vi "DHE_TPs2DArrr.vi"(10 "TPs":T1[](array[typedef]) {"Limits"."nominal" format="%.2f"; "Limits"."Lower" format="%.2f"; "Limits"."upper" format="%.2f"}) -> (2 "TPs out":string[][](table))   [LabVIEW 2016]
uses:
  DHE_TP.ctl
  DHE_TPLimits.ctl
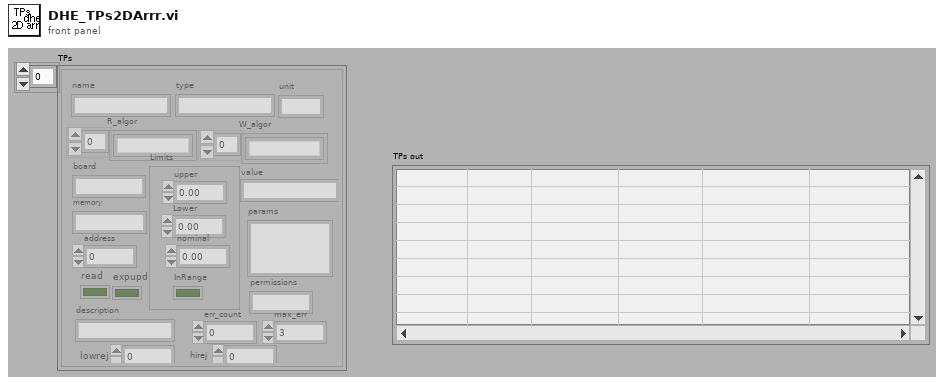
[diagram p1: front panel]
types:
  T1 = typedef "DHE_TP.ctl" = cluster{"name":string, "type":string, "R_algor":string[], "board":string, "memory":string, "address":i32, "value":string, "Limits":T2, "unit":string, "params":string, "permissions":string, "W_algor":string[], "description":string, "err_count":i32, "max_err":i32, "read":bool, "lowrej":dbl, "hirej":dbl, "expupd":bool}
  T2 = typedef "DHE_TPLimits.ctl" = cluster{"upper":dbl, "Lower":dbl, "InRange":bool, "nominal":dbl}
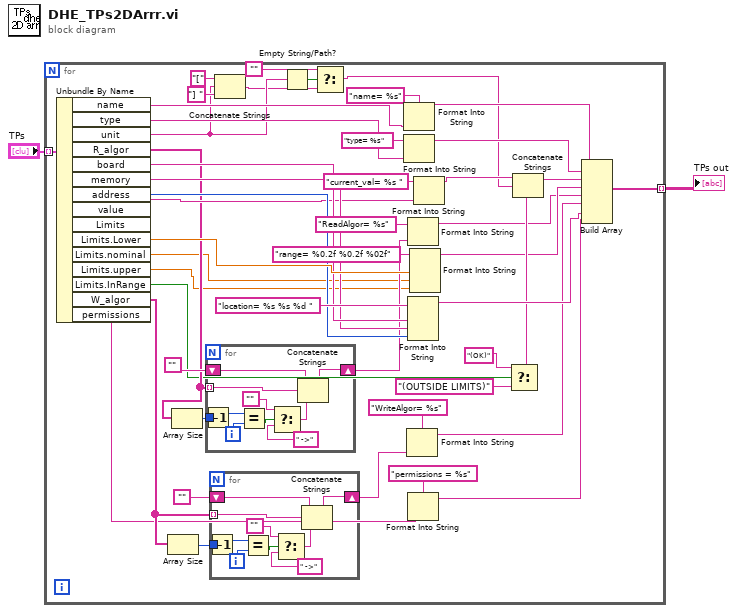
[diagram p0: block diagram]
diagram:
  n1 = for {
    tunnel: "TPs" -> [w50] mode=indexing
    tunnel: [w33] -> w1 mode=indexing
    n2 = Unbundle By Name(w50) -> ("name"=w48:string, "type"=w46:string, "unit"=w21:string, "R_algor"=w31:string[], "board"=w41:string, "memory"=w40:string, "address"=w39:i32, "value"=w37:string, "Limits.Lower"=w43:dbl, "Limits.nominal"=w4:dbl, "Limits.upper"=w5:dbl, "Limits.InRange"=w19:bool, "W_algor"=w12:string[], "permissions"=w7:string)  [unwired: 1 out]
    n3 = Array Size(array=w12) -> (size(s)=w13:i32)
    n4 = Array Size(array=w31) -> (size(s)=w30:i32)
    n5 = for {
      tunnel: w31 -> [w70] mode=indexing
      shift-right: [w69] -> w29
      shift-left: "" -> [w68]
      tunnel: w30 -> [w67]
      i -> [w66]
      n6 = Decrement(x=w67) -> (x-1=w61:i32)
      n7 = Equal?(x=w61, y=w66) -> (x = y?=w65:bool)
      n8 = Select(t="", s=w65, f=" ->") -> (s? t:f=w62:string)
      n9 = Concatenate Strings(w68, w70, w62) -> (w69:string)
    }
    n10 = for {
      tunnel: w12 -> [w60] mode=indexing
      shift-right: [w59] -> w10
      shift-left: "" -> [w58]
      tunnel: w13 -> [w57]
      i -> [w56]
      n11 = Decrement(x=w57) -> (x-1=w51:i32)
      n12 = Equal?(x=w51, y=w56) -> (x = y?=w55:bool)
      n13 = Select(t="", s=w55, f=" ->") -> (s? t:f=w52:string)
      n14 = Concatenate Strings(w58, w60, w52) -> (w59:string)
    }
    n15 = Concatenate Strings("[" ("string"), w21, "] " ("string")) -> (w20:string)
    n16 = Empty String/Path?(string/path=w21) -> (empty?=w28:bool)
    n17 = Select(t="", s=w28, f=w20) -> (s? t:f=w25:string)
    n18 = Format Into String(format string="name= %s", w48) -> (resulting string=w36:string)  [unwired: 2 in, 1 out]
    n19 = Format Into String(format string="type= %s", w46) -> (resulting string=w35:string)  [unwired: 2 in, 1 out]
    n20 = Format Into String(format string="WriteAlgor= %s", w10) -> (resulting string=w9:string)  [unwired: 2 in, 1 out]
    n21 = Format Into String(format string="ReadAlgor= %s", w29) -> (resulting string=w14:string)  [unwired: 2 in, 1 out]
    n22 = Format Into String(format string="location= %s %s %d ", w41, w40, w39) -> (resulting string=w34:string)  [unwired: 2 in, 1 out]
    n23 = Format Into String(format string="permissions = %s", w7) -> (resulting string=w6:string)  [unwired: 2 in, 1 out]
    n24 = Format Into String(format string="range= %0.2f %0.2f %02f", w43, w4, w5) -> (resulting string=w15:string)  [unwired: 2 in, 1 out]
    n25 = Format Into String(format string="current_val= %s ", w37) -> (resulting string=w26:string)  [unwired: 2 in, 1 out]
    n26 = Select(t="(OK)", s=w19, f="(OUTSIDE LIMITS)") -> (s? t:f=w16:string)
    n27 = Concatenate Strings(w26, w25, w16) -> (w24:string)
    n28 = Build Array(w36, w35, w24, w15, w14, w9, w34, w6) -> (w33:string[])
  }
  "TPs out" <- w1
